vi "FdxFwIrig2StructIrigCvi.vi"(8 "error in":errorcluster, 11 "FwIrigTime":cluster{"TtHigh":u32, "TtLow":u32}) -> (0 "error out":errorcluster, 1 "IrigTime":T1)   [LabVIEW 2020, in "AIM664LV.lvlib"]
doc: "This function can be used to convert an IRIG time in the format used by the Firmware to a structured format. This function is helpful since the format of the IRIG time used by the firmware is different to the format often used in the Application Library."
uses:
  AIM664LV.lvlib
  AFDX_Controls/IrigTime.ctl
  AFDX_LibraryAdmin/FdxGlobalDllPath.vi
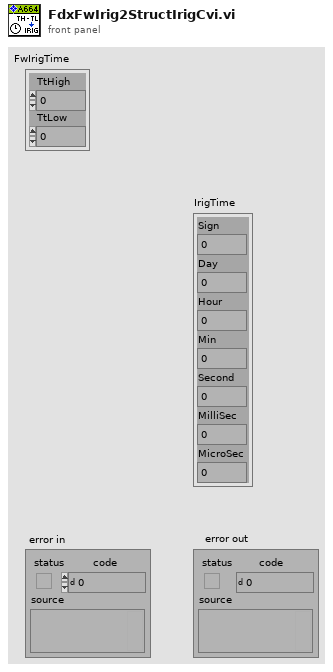
[diagram p1: front panel]
types:
  T1 = typedef "AIM664LV.lvlib/IrigTime.ctl" = cluster{"Sign":i32, "Day":u32, "Hour":u32, "Min":u32, "Second":u32, "MilliSec":u32, "MicroSec":u32}
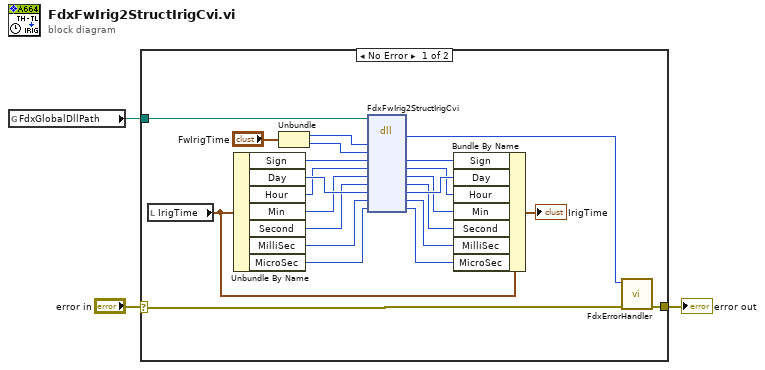
[diagram p0: block diagram]
diagram:
  n1 = global read "FdxGlobalDllPath.vi" "FdxGlobalDllPath"() -> (w1:path)
  n2 = case shown="No Error" "error in" {
    selector: "error in" -> [w25 w27]
    tunnel: [w26 w27] -> w3
    tunnel: w1 -> [w12 _]
    frame No Error {
      n3 = local read "IrigTime"() -> (w15:T1)
      n4 = Unbundle By Name(w15) -> ("Sign"=w18:i32, "Day"=w11:u32, "Hour"=w9:u32, "Min"=w8:u32, "Second"=w7:u32, "MilliSec"=w17:u32, "MicroSec"=w16:u32)
      n5 = Unbundle("FwIrigTime") -> ("TtHigh"=w21:u32, "TtLow"=w20:u32)
      n6 = dll-call lib="aim_fdx.19.dll" fn="FdxFwIrig2StructIrigCvi"(path in=w12, "TtHigh"=w21, "TtLow"=w20, "Sign"=w18, "Hour"=w9, "Min"=w8, "Second"=w7, "Day"=w11, "MilliSec"=w17, "MicroSec"=w16) -> ("status"=w24:i32, "Sign"=w19:i32, "Hour"=w6:u32, "Min"=w5:u32, "Second"=w4:u32, "Day"=w10:u32, "MilliSec"=w14:u32, "MicroSec"=w13:u32)  [unwired: 4 in, 2 out]
      n7 = Bundle By Name(cluster=w15, "Sign"=w19, "Day"=w10, "Hour"=w6, "Min"=w5, "Second"=w4, "MilliSec"=w14, "MicroSec"=w13) -> (→"IrigTime":T1)
      n8 = call "FdxErrorHandler.vi"("error in"=w25, "AIM Error"=w24) -> ("error out"=w26:errorcluster)  [unwired: 9 in]
    }
    frame Error {
    }
  }
  "error out" <- w3
